vi "Configure Pre Filter.vi"(7 "lock-in.prefilter 0":enum16{"1x2SOS", "None", "FIR"}(ring), 8 "error in (no error)":errorcluster, 10 "lock-in.iir config prefilter 0":T1, 11 "LIA Debugging Slow in":refnum<class "LIA Debugging Slow.lvclass">) -> (0 "error out":errorcluster, 3 "LIA Debugging Slow out":refnum<class "LIA Debugging Slow.lvclass">)   [LabVIEW 2017, in "LIA Debugging Slow.lvclass"]
uses:
  LIA Debugging Slow.lvclass
  Shared/lib/interface/Interface FPGA/LIA Host Interface FPGA.lvclass
  Shared/lib/interface/Interface FPGA/Properties/FpgaSession_GET.vi
  <vilib>/Utility/error.llb/Error Cluster From Error Code.vi
  <vilib>/rvi/errors/niLvFpgaAdjustHostInterfaceError.vi
  <vilib>/rvi/interface/nirviReadWriteControl/nirviReadWriteControl.xnode
  NiFpgaLv.dll
  <vilib>/rvi/interface/Simulation/niFpgaSimulationCallBeginRW.vi
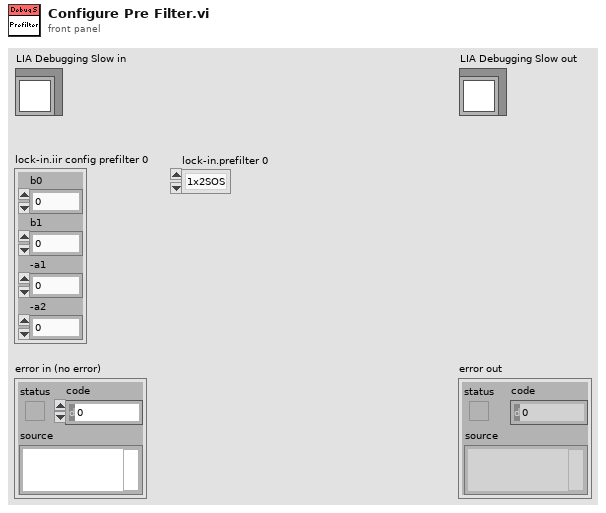
[diagram p1: front panel]
types:
  T1 = cluster{"b0":fxp<+/-,18,2>, "b1":fxp<+/-,18,2>, "-a1":fxp<+/-,18,2>, "-a2":fxp<+/-,18,2>}
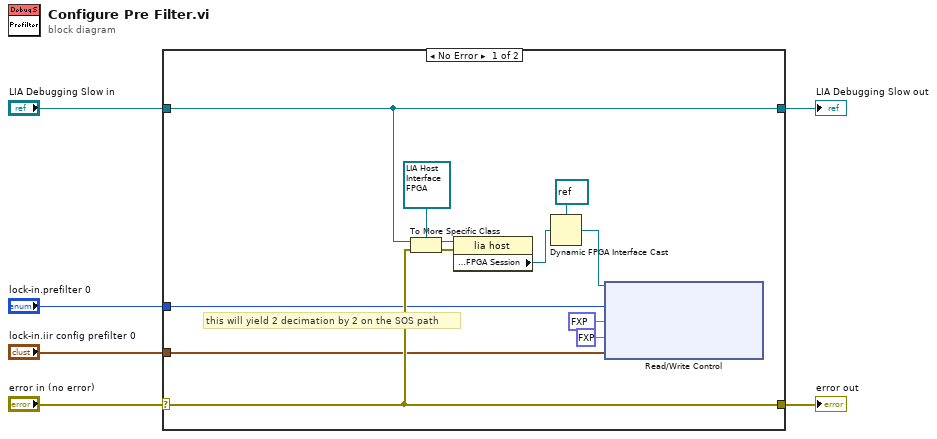
[diagram p0: block diagram]
diagram:
  n1 = case shown="No Error" "error in (no error)" {
    selector: "error in (no error)" -> [w12 w20]
    tunnel: [w12 w20] -> w5
    tunnel: [w13 w19] -> w3
    tunnel: "LIA Debugging Slow in" -> [w13 w19]
    tunnel: "lock-in.iir config prefilter 0" -> [w8 _]
    tunnel: "lock-in.prefilter 0" -> [w7 _]
    frame No Error {
      # "this will yield 2 decimation by 2 on the SOS path"
      n2 = To More Specific Class(target class=refnum<class "LIA Host Interface FPGA.lvclass"> refnum ("lia host"), reference=w13, error in=w12) -> (specific class reference=w16:refnum<class "LIA Host Interface FPGA.lvclass">, error out=w15:errorcluster)
      n3 = property class="lia host"(reference=w16, error in=w15) -> ("Properties:FPGA Session"=w17:refnum<k20>)  [unwired: 2 out]
      n4 = Dynamic FPGA Interface Cast(Session In=refnum<k20> refnum ("fpga type"), Type=w17) -> (Session Out=w11:refnum<k20>)
      n5 = xnode "Read/Write Control"("FPGA VI Reference In"=w11, "lock-in.prefilter 0"=w7, "lock-in.fir fs prefilter 0"=fxp<+,48,1> 0.25, "lock-in.iir prefilter 0"=fxp<+,4,4> 1.0 ("lock-in.iir decimation0 0"), "lock-in.iir config prefilter 0"=w8) -> ()  [unwired: 1 in, 2 out]
    }
    frame Error {
    }
  }
  "error out" <- w5
  "LIA Debugging Slow out" <- w3
